vi "cvt_Bool_TagList.vi"(8 "error in (no error)":errorcluster, 9 "Tag Name":string, 10 "Tag List":T1[](array[typedef]), 11 "Method":T3=enum."getindex") -> (0 "error out":errorcluster, 1 "Tag Index":i32, 2 "Default Data":bool[](array[boolean]), 3 "Tag Description":string, 5 "Bool Tag List":T1[](array[typedef]))   [LabVIEW 2010]
uses:
  TypeDefs/cvt_TagList Methods.ctl
  TypeDefs/cvt_Tag Configuration.ctl
  TypeDefs/cvt_Data Types.ctl
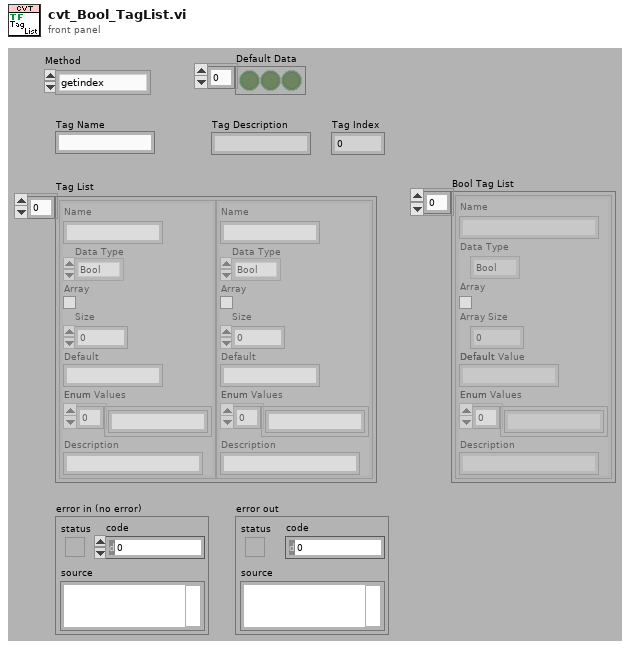
[diagram p1: front panel]
types:
  T1 = typedef "cvt_Tag Configuration.ctl" = cluster{"Name":string, "Data Type":T2, "Array":bool, "Size":u32, "Default":string, "Enum":string[], "Description":string}
  T2 = typedef "cvt_Data Types.ctl" = enum16{"Bool", "U8", "I32", "Double", "String", "Enum"}
  T3 = typedef "cvt_TagList Methods.ctl" = enum16{"init", "getindex", "getdesc", "getlist"}
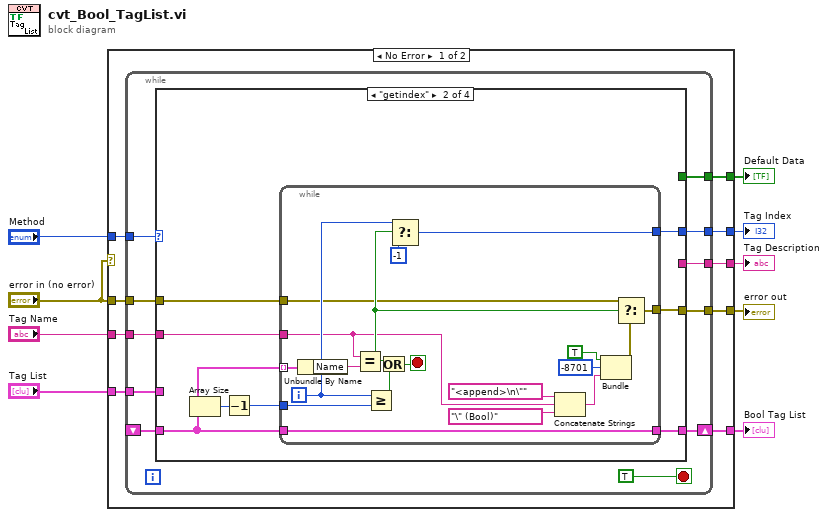
[diagram p0: block diagram]
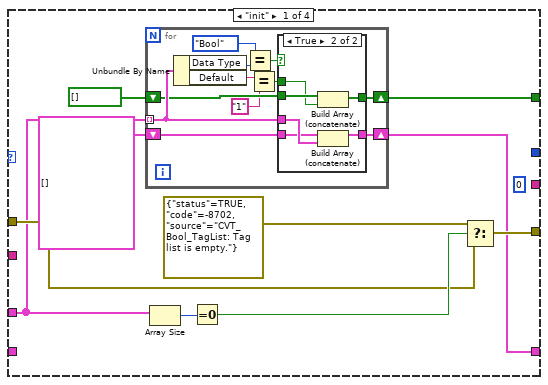
[diagram p2: hidden frame]
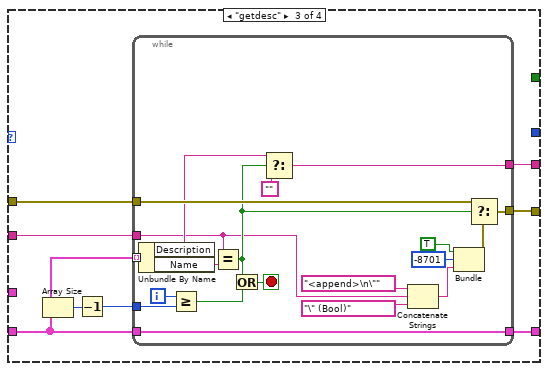
[diagram p4: hidden frame]
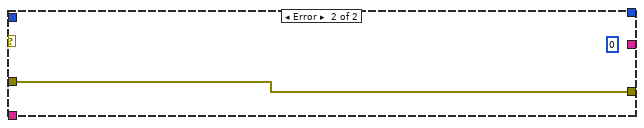
[diagram p6: hidden frame]
diagram:
  n1 = case shown="No Error" "error in (no error)" {
    tunnel: "Method" -> [w18 _]
    tunnel: "Tag Name" -> [w17 _]
    tunnel: [w16 w116] -> w7
    tunnel: "error in (no error)" -> [w15 w116]
    tunnel: "Tag List" -> [w14 _]
    tunnel: [w13 _] -> w4
    tunnel: [w12 _] -> w3
    tunnel: [w11 _] -> w2
    tunnel: [w10 _] -> w1
    frame No Error {
      n2 = while {
        tunnel: w18 -> [w28]
        tunnel: w17 -> [w27]
        tunnel: w15 -> [w26]
        tunnel: [w25] -> w16
        tunnel: w14 -> [w22]
        shift-right: [w24] -> w10
        shift-left: _ -> [w23]
        tunnel: [w21] -> w13
        tunnel: [w20] -> w12
        tunnel: [w19] -> w11
        stop <- TRUE stop-if-true
        n3 = case shown="\"getindex\"" w28 {
          tunnel: w27 -> [_ w66 w93 _]
          tunnel: w26 -> [w36 w60 w87 w114]
          tunnel: [w38 w61 w88 w114] -> w25
          tunnel: [w32 w63 w90 w115] -> w24
          tunnel: w23 -> [_ w62 w89 w115]
          tunnel: w22 -> [w33 _ _ _]
          tunnel: [w31 _ _ _] -> w21
          tunnel: [_ _ w86 _] -> w20
          tunnel: [_ w59 _ _] -> w19
          frame "init" {
            (unwired) 0 ("f")
            n4 = for {
              tunnel: w33 -> [w47] mode=indexing
              shift-right: [w45] -> w32
              shift-left: T1[] [] -> [w46]
              shift-right: [w43] -> w31
              shift-left: bool[] [] -> [w44]
              n5 = Unbundle By Name(w47) -> ("Data Type"=w50:T2, "Default"=w42:string)
              n6 = Equal?(x=cvt_Data_Types."Bool", y=w50) -> (x = y?=w49:bool)
              n7 = Equal?(x=w42, y="1") -> (x = y?=w41:bool)
              n8 = case shown="True" w49 {
                tunnel: w44 -> [w51 w58]
                tunnel: [w51 w57] -> w43
                tunnel: w47 -> [_ w56]
                tunnel: w46 -> [w52 w55]
                tunnel: [w52 w54] -> w45
                tunnel: w41 -> [_ w53]
                frame False {
                }
                frame True {
                  n9 = Build Array (concatenate)(w58, w53) -> (w57:bool[])
                  n10 = Build Array (concatenate)(w55, w56) -> (w54:T1[])
                }
              }
            }
            n11 = Array Size(array=w33) -> (size(s)=w39:i32)
            n12 = Equal To 0?(x=w39) -> (x = 0?=w37:bool)
            n13 = Select(t=errorcluster {"status"=TRUE, "code"=-8702, "source"="CVT_Bool_TagList: Tag list is empty."} ("f"), s=w37, f=w36) -> (s? t:f=w38:errorcluster)
          }
          frame "getindex" {
            n14 = Array Size(array=w62) -> (size(s)=w65:i32)
            n15 = Decrement(x=w65) -> (x-1=w64:i32)
            n16 = while {
              tunnel: w62 -> [w85] mode=indexing
              tunnel: w66 -> [w70]
              tunnel: w64 -> [w83]
              tunnel: [w74] -> w59
              tunnel: [w77] -> w63
              tunnel: w62 -> [w77]
              tunnel: [w76] -> w61
              tunnel: w60 -> [w75]
              i -> [w80]
              stop <- w81 stop-if-true
              n17 = Unbundle By Name(w85) -> ("Name"=w84:string)
              n18 = Equal?(x=w70, y=w84) -> (x = y?=w78:bool)
              n19 = Greater Or Equal?(x=w80, y=w83) -> (x >= y?=w82:bool)
              n20 = Or(x=w78, y=w82) -> (x .or. y?=w81:bool)
              n21 = Select(t=w80, s=w78, f=-1) -> (s? t:f=w74:i32)
              n22 = Concatenate Strings("<append>\n\"" ("source"), w70, "\" (Bool)" ("source")) -> (w69:string)
              n23 = Bundle("status"=TRUE, "code"=-8701, w69) -> (w68:cluster{"status":bool, "code":i32, string})  [unwired: 1 out]
              n24 = Select(t=w75, s=w78, f=w68) -> (s? t:f=w76:errorcluster)
            }
          }
          frame "getdesc" {
            n25 = Array Size(array=w89) -> (size(s)=w92:i32)
            n26 = Decrement(x=w92) -> (x-1=w91:i32)
            n27 = while {
              tunnel: w89 -> [w113] mode=indexing
              tunnel: w93 -> [w94]
              tunnel: w91 -> [w111]
              tunnel: [w103] -> w86
              tunnel: [w107] -> w90
              tunnel: w89 -> [w107]
              tunnel: [w106] -> w88
              tunnel: w87 -> [w105]
              i -> [w108]
              stop <- w109 stop-if-true
              n28 = Unbundle By Name(w113) -> ("Description"=w102:string, "Name"=w112:string)
              n29 = Greater Or Equal?(x=w108, y=w111) -> (x >= y?=w110:bool)
              n30 = Equal?(x=w94, y=w112) -> (x = y?=w101:bool)
              n31 = Or(x=w101, y=w110) -> (x .or. y?=w109:bool)
              n32 = Select(t=w102, s=w101, f="") -> (s? t:f=w103:string)
              n33 = Concatenate Strings("<append>\n\"" ("source"), w94, "\" (Bool)" ("source")) -> (w97:string)
              n34 = Bundle("status"=TRUE, "code"=-8701, w97) -> (w95:cluster{"status":bool, "code":i32, string})  [unwired: 1 out]
              n35 = Select(t=w105, s=w101, f=w95) -> (s? t:f=w106:errorcluster)
            }
          }
          frame "getlist" {
          }
        }
      }
    }
    frame Error {
      (unwired) 0 ("f")
    }
  }
  "error out" <- w7
  "Default Data" <- w4
  "Tag Description" <- w3
  "Tag Index" <- w2
  "Bool Tag List" <- w1
